vi "Untitled 1.vi"() -> ()   [LabVIEW 2016]
uses:
  TTA_Control_RFIC_List.ctl
panel:
  in  "Ring 3":u16(ring)
  in  "Color Box 3":u32(colorbox)
  in  "Color Box 2":u32(colorbox)
  in  "Color Box":u32(colorbox)
  in  "Ring 2":u16(ring)
  in  "Ring":u16(ring) items=["Complete", "Failed", "Running..."]
  in  "stop":bool
  out "error out":errorcluster
  in  "error in (no error)":errorcluster
  out "Value":T1 caption="RFIC List"
  in  "RFIC List":T2(array[cluster])
  # "Test Description"
  # "Enable"
  # "Channel 1"
  # "Channel 2"
  # "FAILED"
  # "Running..."
  # "PASSED"
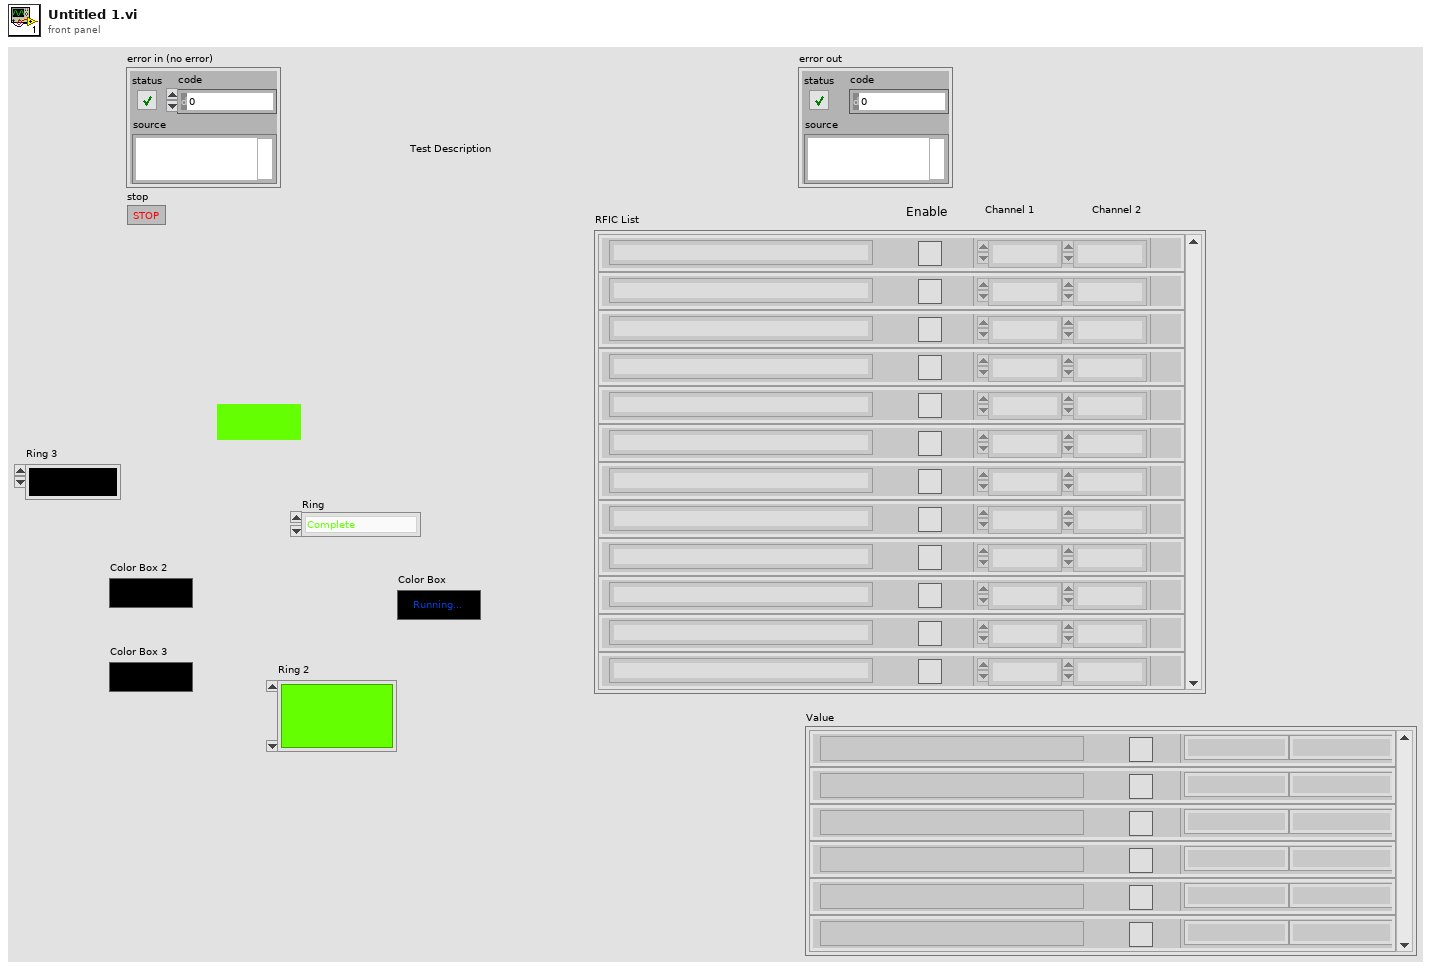
[diagram p1: front panel]
types:
  T1 = typedef "TTA_Control_RFIC_List.ctl" = cluster{"Enable":bool, "Test Description":string, "Array":string[]}[]
  T2 = cluster{"Enable":bool, "Test Description":string, "Array":u16[]}[]
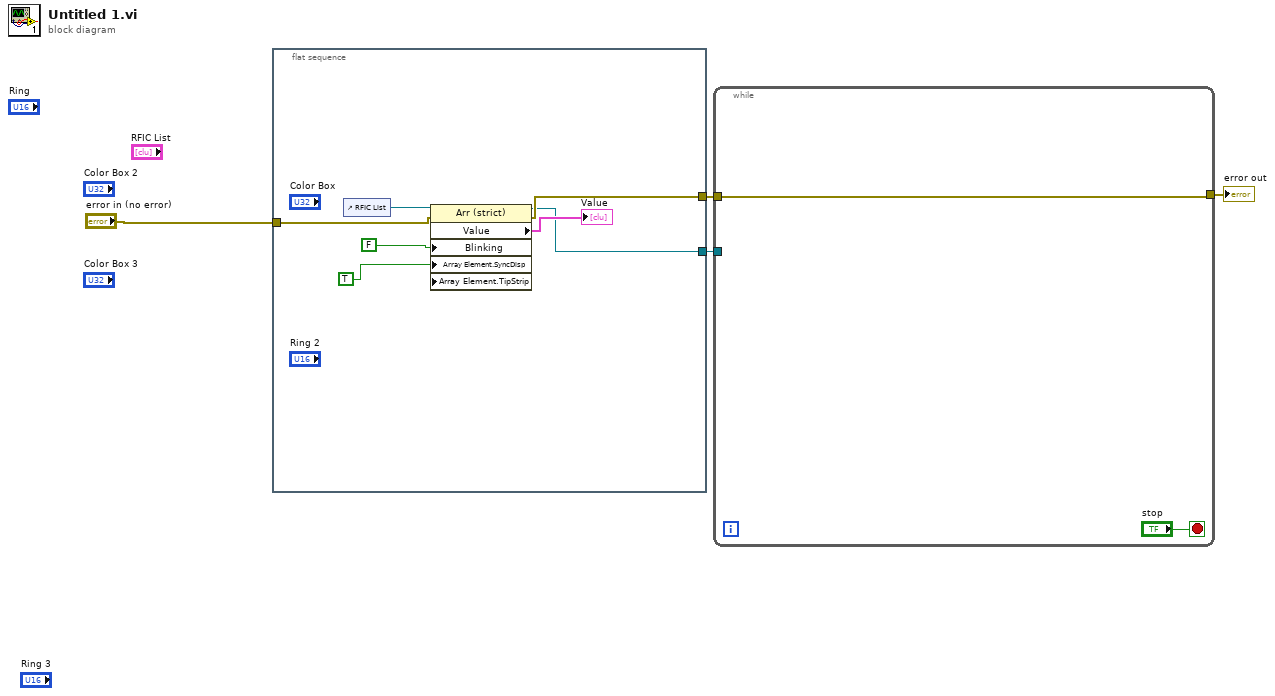
[diagram p0: block diagram]
diagram:
  n1 = flat-sequence {
    tunnel: [w9] -> w4
    tunnel: "error in (no error)" -> [w8]
    tunnel: [w6] -> w1
    frame #0 {
      n2 = control-ref of="RFIC List"() -> (w11:refnum<vi>)
      n3 = property class="Arr (strict)" props=["Value", "Blinking", "Array Element", "SyncDisp", "Array Element", "TipStrip"](reference=w11, error in=w8, "Blinking"=FALSE, "Array Element.SyncDisp"=TRUE ("Array Element.Synchronous Display")) -> (reference out=w6:refnum<vi>, error out=w9:errorcluster, "Value"=→"Value":T2)  [unwired: 1 in]
    }
  }
  n4 = while {
    tunnel: w4 -> [w13]
    tunnel: [w13] -> w3
    tunnel: w1 -> [_]
    stop <- "stop" stop-if-true
  }
  "error out" <- w3
